vi "counting7segDisplay.vi"() -> ()   [LabVIEW 2015]
panel:
  in  "Stop Button":bool
  out "error out 5":errorcluster
  in  "task/channels in 2":refnum<k21>
  in  "Count Up or Down?":bool
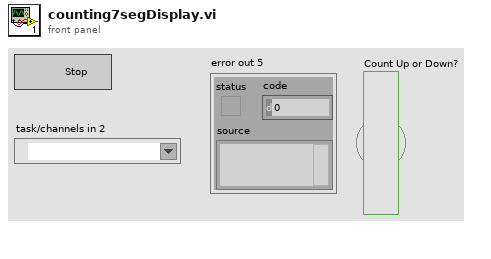
[diagram p1: front panel]
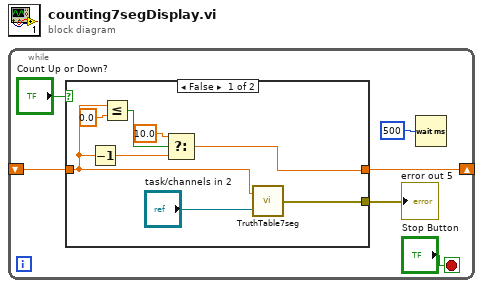
[diagram p0: block diagram]
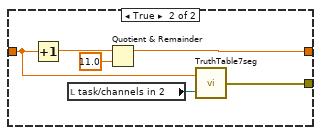
[diagram p2: hidden frame]
diagram:
  n1 = while {
    shift-right: [w2] -> _
    shift-left: _ -> [w1]
    stop <- "Stop Button" stop-if-true
    n2 = case shown="False" "Count Up or Down?" {
      tunnel: [w14 w19] -> w4
      tunnel: [w12 w18] -> w2
      tunnel: w1 -> [w7 w15]
      frame False {
        n3 = Decrement(x=w7) -> (x-1=w10:dbl)
        n4 = Less Or Equal?(x=w7, y=0.0) -> (x <= y?=w9:bool)
        n5 = Select(t=10.0, s=w9, f=w10) -> (s? t:f=w12:dbl)
        n6 = call "TruthTable7seg.vi"("task/channels in"="task/channels in 2", "Numeric Control"=w7) -> ("error out 2"=w14:errorcluster)
      }
      frame True {
        n7 = Increment(x=w15) -> (x+1=w16:dbl)
        n8 = local read "task/channels in 2"() -> (w20:refnum<k21>)
        n9 = Quotient & Remainder(x=w16, y=11.0) -> (x-y*floor(x/y)=w18:dbl)  [unwired: 1 out]
        n10 = call "TruthTable7seg.vi"("task/channels in"=w20, "Numeric Control"=w15) -> ("error out 2"=w19:errorcluster)
      }
    }
    "error out 5" <- w4
    n11 = Wait (ms)(milliseconds to wait=u32 500) -> ()  [unwired: 1 out]
  }
